vi "Prompt for Step--UI Interlocks.vi"(8 "error in (no error)":errorcluster, 10 "Control Ref Map":map{string, refnum<vi>}(c390), 11 "Timing Action in":refnum<class "Timing Action.lvclass">) -> (0 "error out":errorcluster, 2 "Error List":string[](array[string]), 3 "Timing Action out":refnum<class "Timing Action.lvclass">)   [LabVIEW 2020, in "MacroAssert.lvlib" / "Timing Action.lvclass"]
doc: "Enables or disables buttons within the \"Prompt for Step\" VI according to the current state of the system."
uses:
  Timing Action.lvclass
  Timing Action Type.ctl
  Support/Get Control Reference by Label (1D STR).vi
  MacroAssert.lvlib
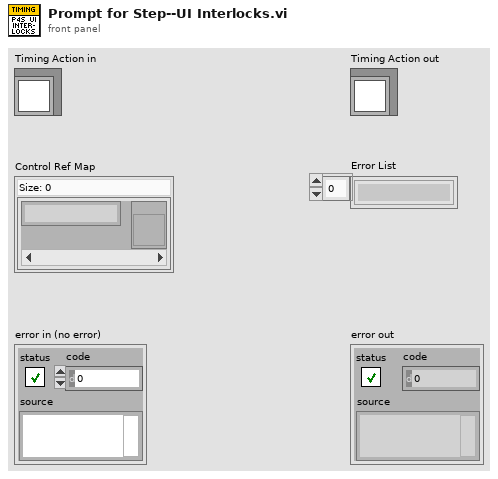
[diagram p1: front panel]
types:
  T1 = typedef "MacroAssert.lvlib/Timing Action.lvclass/Timing Action Type.ctl" = enum16{"Wait", "Wait Until"}
  T2 = enum8{"Enabled", "Disabled", "Disabled and Grayed Out"}
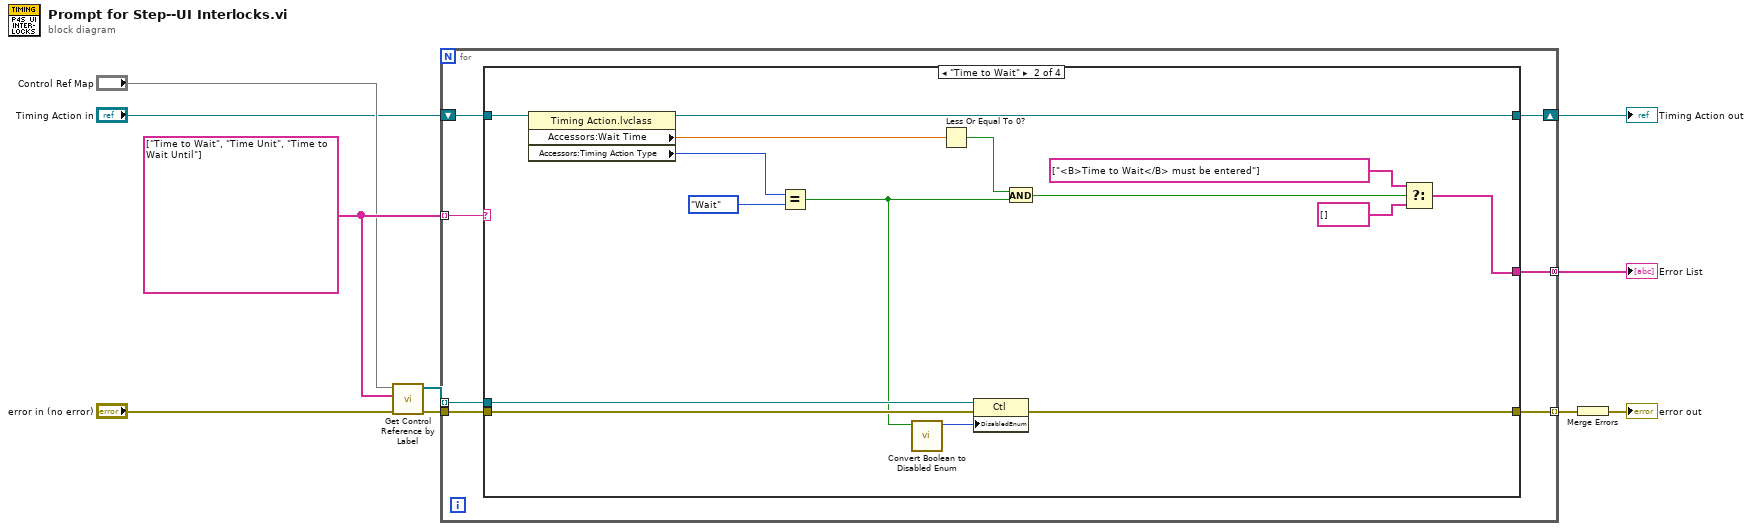
[diagram p0: block diagram]
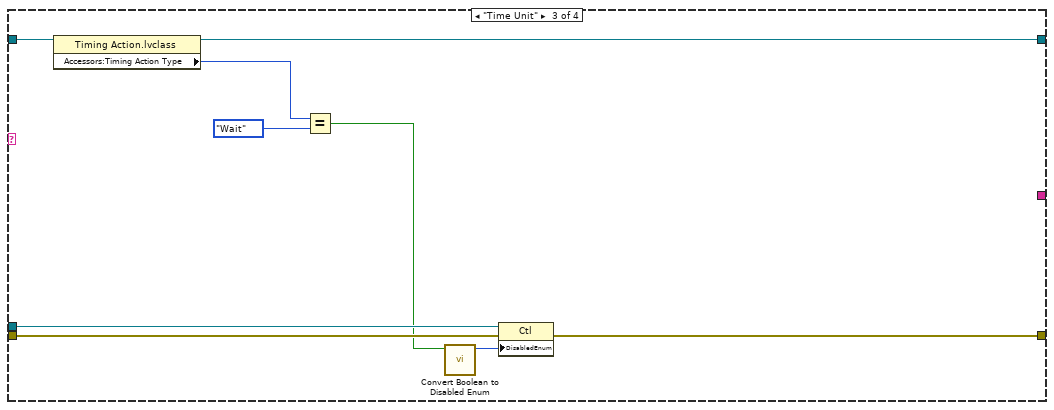
[diagram p3: hidden frame]
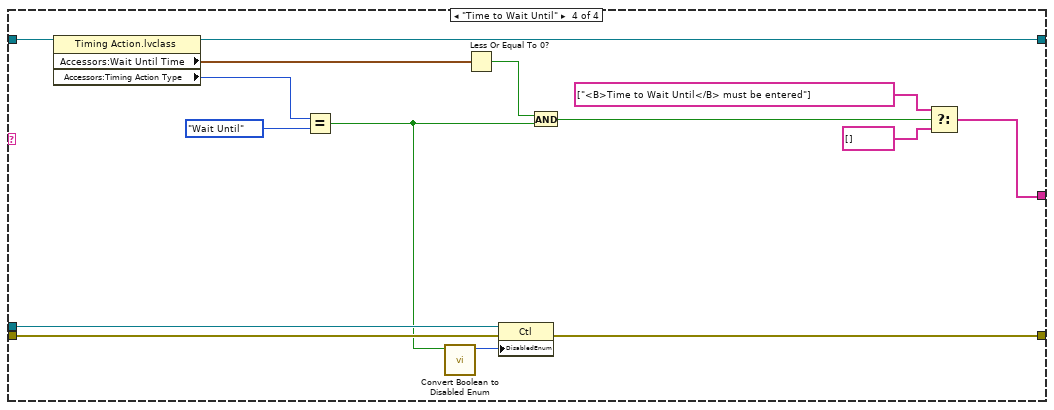
[diagram p4: hidden frame]
diagram:
  w8 = string[] ["Time to Wait", "Time Unit", "Time to Wait Until"]
  n1 = call-poly "Get Control Reference by Label.vi"("error in (no error)"="error in (no error)", "Control Names"=w8, "Control Ref Map"="Control Ref Map") -> ("error out"=w10:errorcluster, "Control Refs"=w9:refnum<vi>[])  [unwired: 6 in, 1 out]
  n2 = for {
    shift-right: [w14] -> w2
    shift-left: "Timing Action in" -> [w17]
    tunnel: w8 -> [w16] mode=indexing
    tunnel: [w15] -> w7 mode=indexing
    tunnel: w10 -> [w13]
    tunnel: w9 -> [w12] mode=indexing
    tunnel: [w11] -> w1 mode=concatenating
    n3 = case shown="\"Time to Wait\"" w16 {
      tunnel: w17 -> [w18 w34 w43 w58]
      tunnel: w13 -> [w19 w32 w41 w56]
      tunnel: [w19 w24 w38 w48] -> w15
      tunnel: [w18 w33 w42 w57] -> w14
      tunnel: w12 -> [_ w23 w37 w47]
      tunnel: [_ w29 _ w53] -> w11
      frame Default {
      }
      frame "Time to Wait" {
        n4 = property class="Timing Action.lvclass"(reference=w34) -> (reference out=w33:refnum<class "Timing Action.lvclass">, "Accessors:Wait Time"=w28:dbl, "Accessors:Timing Action Type"=w26:T1)  [unwired: 1 in, 1 out]
        n5 = Equal?(x=w26, y=Timing_Action_Type."Wait") -> (x = y?=w20:bool)
        n6 = call "Convert Boolean to Disabled Enum.vi"("Enabled?"=w20) -> ("Disabled Enum"=w22:T2)  [unwired: 10 in]
        n7 = Less Or Equal To 0?(x=w28) -> (x <= 0?=w27:bool)
        n8 = property class="Ctl"(reference=w23, error in=w32, "DisabledEnum"=w22) -> (error out=w24:errorcluster)  [unwired: 1 out]
        n9 = And(x=w27, y=w20) -> (x .and. y?=w21:bool)
        n10 = Select(t=string[] ["<B>Time to Wait</B> must be entered"], s=w21, f=string[] []) -> (s? t:f=w29:string[])
      }
      frame "Time Unit" {
        n11 = property class="Timing Action.lvclass"(reference=w43) -> (reference out=w42:refnum<class "Timing Action.lvclass">, "Accessors:Timing Action Type"=w40:T1)  [unwired: 1 in, 1 out]
        n12 = Equal?(x=w40, y=Timing_Action_Type."Wait") -> (x = y?=w35:bool)
        n13 = call "Convert Boolean to Disabled Enum.vi"("Enabled?"=w35) -> ("Disabled Enum"=w36:T2)  [unwired: 10 in]
        n14 = property class="Ctl"(reference=w37, error in=w41, "DisabledEnum"=w36) -> (error out=w38:errorcluster)  [unwired: 1 out]
      }
      frame "Time to Wait Until" {
        n15 = property class="Timing Action.lvclass"(reference=w58) -> (reference out=w57:refnum<class "Timing Action.lvclass">, "Accessors:Wait Until Time"=w52:timestamp, "Accessors:Timing Action Type"=w50:T1)  [unwired: 1 in, 1 out]
        n16 = Equal?(x=w50, y=Timing_Action_Type."Wait Until") -> (x = y?=w44:bool)
        n17 = call "Convert Boolean to Disabled Enum.vi"("Enabled?"=w44) -> ("Disabled Enum"=w46:T2)  [unwired: 10 in]
        n18 = Less Or Equal To 0?(x=w52) -> (x <= 0?=w51:bool)
        n19 = property class="Ctl"(reference=w47, error in=w56, "DisabledEnum"=w46) -> (error out=w48:errorcluster)  [unwired: 1 out]
        n20 = And(x=w51, y=w44) -> (x .and. y?=w45:bool)
        n21 = Select(t=string[] ["<B>Time to Wait Until</B> must be entered"], s=w45, f=string[] []) -> (s? t:f=w53:string[])
      }
    }
  }
  "Timing Action out" <- w2
  "Error List" <- w1
  n22 = Merge Errors(w7) -> (→"error out":errorcluster)
